vi "Check Sudoku Integer.vi"(8 "error in (no error)":errorcluster, 11 "Sudoku Class in":refnum<class "Sudoku Class.lvclass">) -> (0 "error out":errorcluster, 2 "Is Ok":bool, 3 "Sudoku Class out":refnum<class "Sudoku Class.lvclass">)   [LabVIEW 2015, in "Sudoku Library.lvlib" / "Sudoku Class.lvclass"]
doc: "Created IvanLis by LabVIEW Portal\nProfile: http://labviewportal.org/memberlist.php?mode=viewprofile&u=987\neMail: IvanLisanov@gMail.com\nTelegram: https://t.me/IvanLis"
uses:
  Sudoku Class.lvclass
  Sudoku Class.lvclass/Sudoku Class.ctl
  Sudoku Library.lvlib
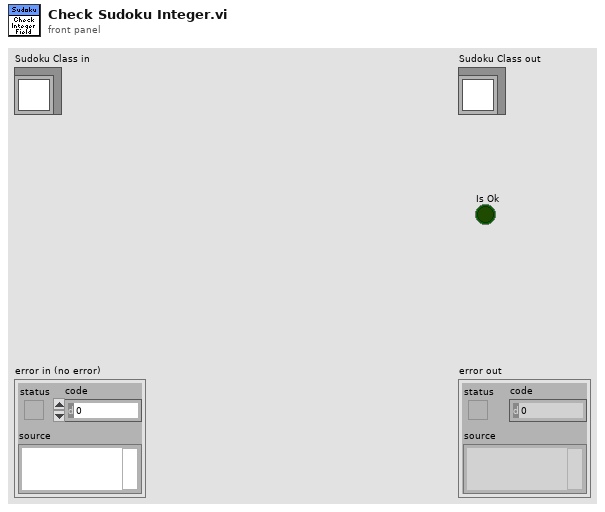
[diagram p1: front panel]
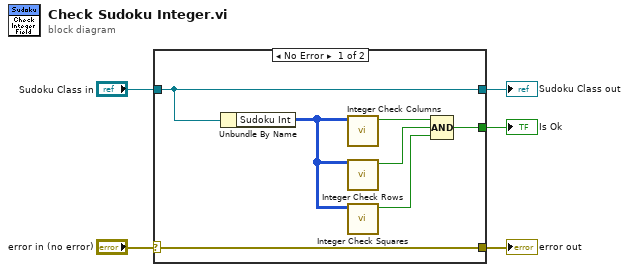
[diagram p0: block diagram]
diagram:
  n1 = case shown="No Error" "error in (no error)" {
    selector: "error in (no error)" -> [w12 w14]
    tunnel: [w12 w14] -> w4
    tunnel: [w11 w13] -> w2
    tunnel: "Sudoku Class in" -> [w11 w13]
    tunnel: [w6 _] -> w1
    frame No Error {
      n2 = Unbundle By Name(w11) -> ("Sudoku Int"=w10:u8[][])
      n3 = call "Integer Check Columns.vi"("Sudoku Int"=w10) -> ("Is Ok"=w9:bool)  [unwired: 10 in]
      n4 = call "Integer Check Rows.vi"("Sudoku Int"=w10) -> ("Is Ok"=w8:bool)  [unwired: 10 in]
      n5 = call "Integer Check Squares.vi"("Sudoku Int"=w10) -> ("Is Ok"=w7:bool)  [unwired: 10 in]
      n6 = Compound Arithmetic op=AND(w9, w8, w7) -> (w6:bool)
    }
    frame Error {
    }
  }
  "error out" <- w4
  "Sudoku Class out" <- w2
  "Is Ok" <- w1
